vi "SignalMeasurements2.vi"() -> ()   [LabVIEW 2025]
uses:
  <vilib>/Waveform/WDTOps.llb/WDT Waveform Duration DBL.vi
  <vilib>/Waveform/WDTOps.llb/WDT Number of Waveform Samples DBL.vi
  <vilib>/measure/NI_MAPro.lvlib
  <vilib>/measure/maspectr.llb/FFT Power Spectrum and PSD for 1 Chan.vi
  <vilib>/Analysis/4window.llb/windowTd.ctl
  <vilib>/Analysis/NI_AALPro.lvlib
panel:
  in  "dB On (F)":bool
  out "error out":errorcluster
  out "number of samples":i32
  out "signal duration":dbl format="%0.2f"
  out "averages completed":dbl
  in  "restart averaging (F)":bool
  in  "window":T1=1 items=["Rectangle"=0, "Hanning"=1, "Hamming"=2, "Blackman-Harris"=3, "Exact Blackman"=4, "Blackman"=5, "Flat Top"=6, "4 Term B-Harris "=7, "7 Term B-Harris"=8, "Low Sidelobe"=9, "Blackman Nuttall"=11, "Triangle"=30, "Bartlett-Hanning"=31, "Bohman"=32, "Parzen"=33, "Welch"=34, "Kaiser"=60, "Dolph-Chebyshev"=61, "Gaussian"=62]
  in  "averaging parameters":T2={"averaging mode"=enum."No averaging", "weighting mode"=enum."Exponential", "number of averages"=10} {"number of averages" min=1}
  in  "error in (no error)":errorcluster
  in  "signal in":waveform(dbl)
  out "frequency domain":cluster{"f0":dbl, "df":dbl, "magnitude":dbl[]}(graph)
  out "time domain":waveform(dbl)(graph)
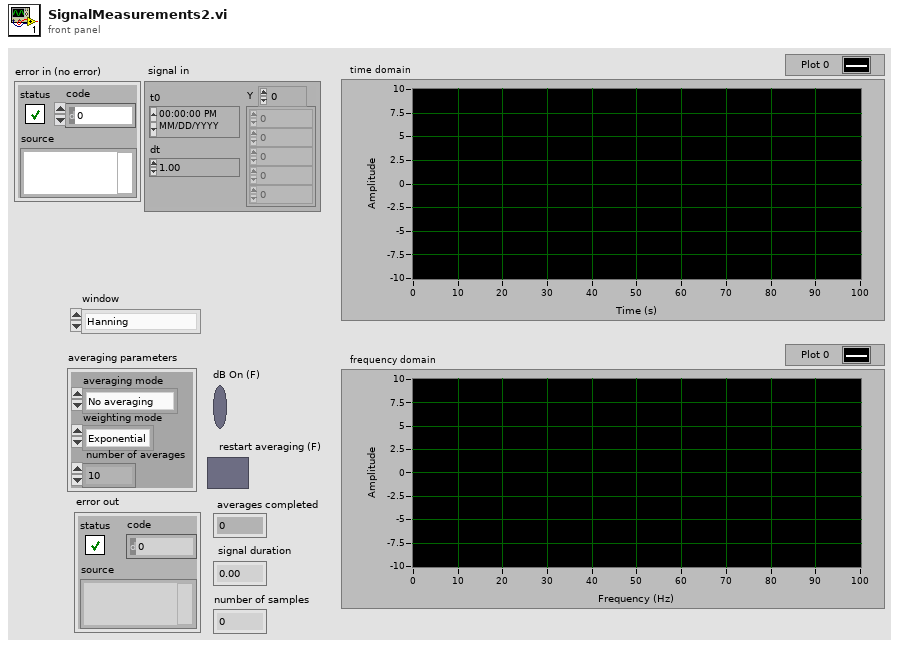
[diagram p1: front panel]
types:
  T1 = typedef "NI_AALPro.lvlib/windowTd.ctl" = u32
  T2 = cluster{"averaging mode":enum16{"No averaging", "Vector averaging", "RMS averaging", "Peak hold"}, "weighting mode":enum16{"Linear", "Exponential"}, "number of averages":u32}
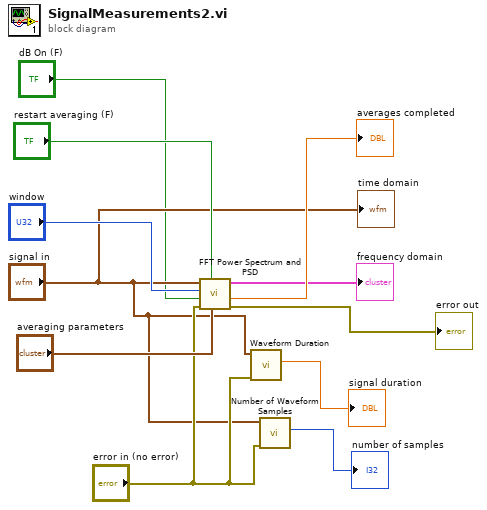
[diagram p0: block diagram]
diagram:
  n1 = call-poly <vilib>:"FFT Power Spectrum and PSD.vi"("averaging parameters"="averaging parameters", "restart averaging (F)"="restart averaging (F)", "error in (no error)"="error in (no error)", "dB On (F)"="dB On (F)", "window"="window", "time signal"="signal in") -> ("error out"=→"error out":errorcluster, "averages completed"=→"averages completed":dbl, "Power Spectrum / PSD"=→"frequency domain":cluster{"f0":dbl, "df":dbl, "magnitude":dbl[]})  [unwired: 2 in, 1 out]
  n2 = call-poly <vilib>:"Waveform Duration.vi"("error in (no error)"="error in (no error)", "waveform in"="signal in") -> ("duration"=→"signal duration":dbl)  [unwired: 7 in, 2 out]
  n3 = call-poly <vilib>:"Number of Waveform Samples.vi"("error in (no error)"="error in (no error)", "waveform in"="signal in") -> ("number of samples"=→"number of samples":i32)  [unwired: 7 in, 2 out]
  "time domain" <- "signal in"
